vi "Create Plugins.vi"(5 "framework options":T1={"FIFO Options"={"Infinite Timeouts"=FALSE}, "Thread Options"={"Show FP On Call"=FALSE, "Close FP After Call"=FALSE, "Allow Debugging"=FALSE}, "Plugin Options"={"Default Components"=FALSE}, "Performance Options"={"Measure Period"=FALSE, "Measure Rx/Tx Duration"=FALSE}, "Data Server Options"={"Enable Data Server"=FALSE, "Period"=50}} {"Data Server Options"."Period" format="%d ms"}, 7 "framework configuration":T7, 8 "error in (no error)":errorcluster, 10 "components directory":path, 11 "Framework in":refnum<class "Framework.lvclass">) -> (0 "error out":errorcluster, 1 "Plugin Threads":refnum<class "Plugin Thread.lvclass">[](array[class]), 2 "Plugins":refnum<class "Plugin.lvclass">[](array[class]), 3 "Framework out":refnum<class "Framework.lvclass">)   [LabVIEW 2017, in "DSF Core.lvlib" / "Framework.lvclass"]
uses:
  Framework.lvclass
  Plugin/Plugin.lvclass
  Typedefs/DSF Engine Framework Configuration.ctl
  Typedefs/DSF Engine Plugin Configuration.ctl
  Typedefs/DSF Timing Info.ctl
  Typedefs/DSF Engine Plugin Thread Configuration.ctl
  Typedefs/DSF Settings Info.ctl
  Typedefs/DSF Engine Transfer Group Configuration.ctl
  Typedefs/DSF Direction.ctl
  Typedefs/DSF Engine Transfer Configuration.ctl
  Typedefs/DSF Byte Order.ctl
  Typedefs/DSF Engine Channel Configuration.ctl
  Typedefs/DSF Data Type.ctl
  Typedefs/DSF Timeout Behavior.ctl
  Thread/Plugin/Plugin Thread.lvclass
  Framework Options.ctl
  Typedefs/DSF FIFO Options.ctl
  Thread/Thread Options.ctl
  Typedefs/DSF Plugin Options.ctl
  Typedefs/DSF Performance Options.ctl
  Data Server Options.ctl
  Transceiver/Transceiver.lvclass
  Buffer Converter/Buffer Converter.lvclass
  Framework.lvclass/Framework.ctl
  Configuration/Transfer Group Count (Plugin).vi
  Configuration/Required Buffer Size (Plugin).vi
  Component Loader/Component Loader.lvclass
  Configuration/Configuration Session.lvclass
  Buffers/Buffers.lvclass
  Status/Status Pointer.lvclass
  Framework Status/Framework Status.lvclass
  DSF Core.lvlib
  Thread/Thread.lvclass
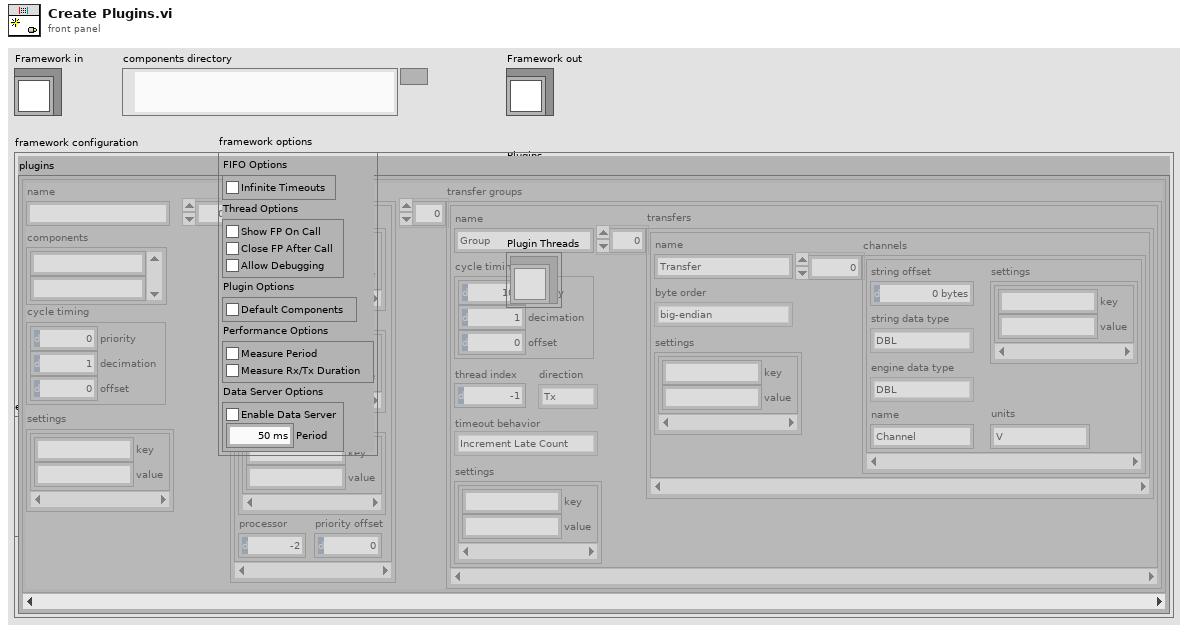
[diagram p1: front panel]
types:
  T1 = typedef "DSF Core.lvlib/Framework.lvclass/Framework Options.ctl" = cluster{"FIFO Options":T2, "Thread Options":T3, "Plugin Options":T4, "Performance Options":T5, "Data Server Options":T6}
  T2 = typedef "DSF Core.lvlib/Framework.lvclass/DSF FIFO Options.ctl" = cluster{"Infinite Timeouts":bool}
  T3 = typedef "DSF Core.lvlib/Thread.lvclass/Thread Options.ctl" = cluster{"Show FP On Call":bool, "Close FP After Call":bool, "Allow Debugging":bool}
  T4 = typedef "DSF Core.lvlib/Framework.lvclass/DSF Plugin Options.ctl" = cluster{"Default Components":bool}
  T5 = typedef "DSF Core.lvlib/DSF Performance Options.ctl" = cluster{"Measure Period":bool, "Measure Rx/Tx Duration":bool}
  T6 = typedef "DSF Core.lvlib/Framework.lvclass/Data Server Options.ctl" = cluster{"Enable Data Server":bool, "Period":u32}
  T7 = typedef "DSF Core.lvlib/DSF Engine Framework Configuration.ctl" = cluster{"plugins":T8[]}
  T8 = typedef "DSF Core.lvlib/DSF Engine Plugin Configuration.ctl" = cluster{"name":string, "components":string[], "cycle timing":T9, "threads":T10[], "transfer groups":T12[], "settings":T11}
  T9 = typedef "DSF Core.lvlib/DSF Timing Info.ctl" = cluster{"priority":u64, "decimation":u64, "offset":u64}
  T10 = typedef "DSF Core.lvlib/DSF Engine Plugin Thread Configuration.ctl" = cluster{"buffer converter settings":T11, "transceiver settings":T11, "custom settings":T11, "processor":i32, "priority offset":i16}
  T11 = typedef "DSF Core.lvlib/DSF Settings Info.ctl" = cluster{"key":string, "value":string}[]
  T12 = typedef "DSF Core.lvlib/DSF Engine Transfer Group Configuration.ctl" = cluster{"name":string, "direction":T13, "cycle timing":T9, "thread index":i32, "settings":T11, "transfers":T14[], "timeout behavior":T18}
  T13 = typedef "DSF Core.lvlib/DSF Direction.ctl" = enum8{"Tx", "Rx"}
  T14 = typedef "DSF Core.lvlib/DSF Engine Transfer Configuration.ctl" = cluster{"name":string, "byte order":T15, "settings":T11, "channels":T16[]}
  T15 = typedef "DSF Core.lvlib/DSF Byte Order.ctl" = enum8{"big-endian", "little-endian"}
  T16 = typedef "DSF Core.lvlib/DSF Engine Channel Configuration.ctl" = cluster{"string offset":u64, "string data type":T17, "engine data type":T17, "name":string, "settings":T11, "units":string}
  T17 = typedef "DSF Core.lvlib/DSF Data Type.ctl" = enum8{"Bool", "SGL", "DBL", "I8", "I16", "I32", "I64", "U8", "U16", "U32", "U64"}
  T18 = typedef "DSF Core.lvlib/DSF Timeout Behavior.ctl" = enum8{"Increment Late Count", "Throw Error"}
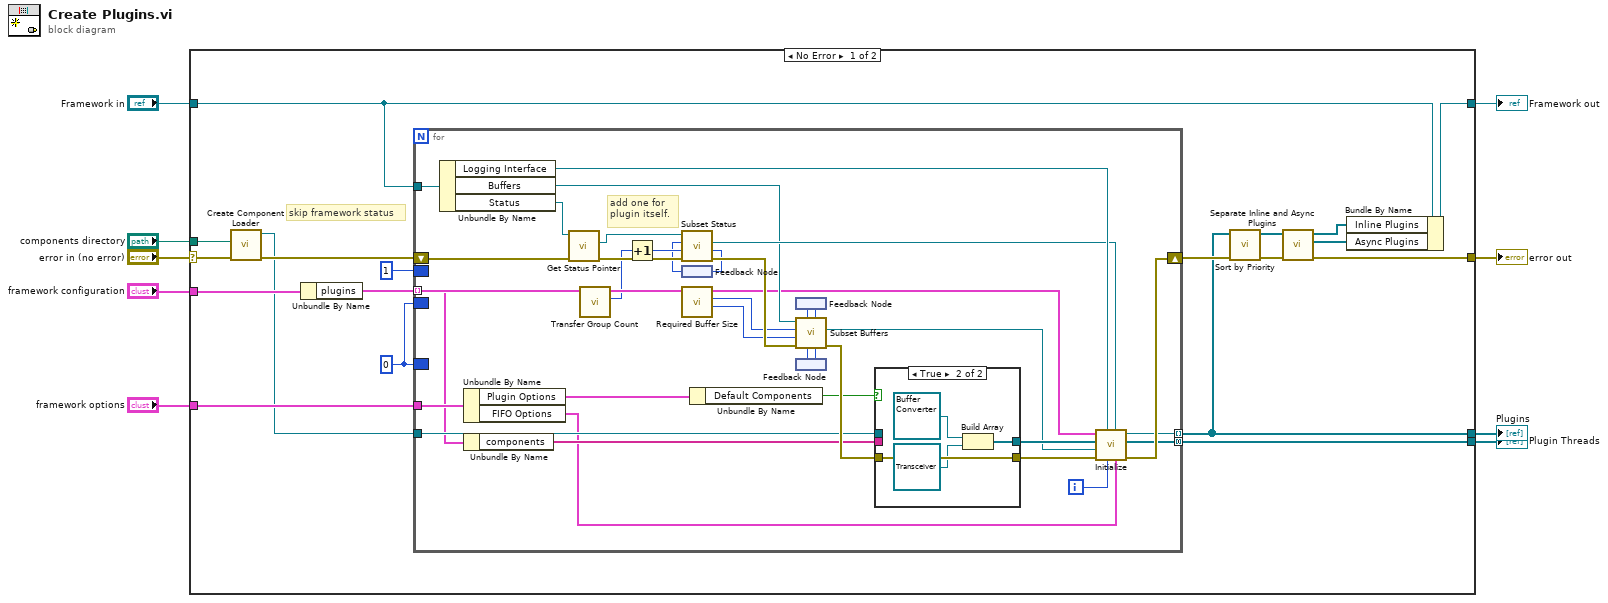
[diagram p0: block diagram]
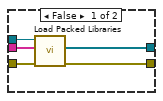
[diagram p2: hidden frame]
diagram:
  n1 = case shown="No Error" "error in (no error)" {
    selector: "error in (no error)" -> [w16 w74]
    tunnel: [w26 w74] -> w9
    tunnel: "framework configuration" -> [w25 _]
    tunnel: [w24 _] -> w7
    tunnel: [w11 _] -> w6
    tunnel: [w20 w75] -> w5
    tunnel: "framework options" -> [w19 _]
    tunnel: "Framework in" -> [w13 w75]
    tunnel: "components directory" -> [w17 _]
    frame No Error {
      w14 = u64 0 ("string buffer offset + size")
      # "skip framework status"
      # "Create Plugins\nIterates through the Plugin configuration clusters to do the following:\n1. Load Plugin components - Uses the Component Loader class to load an array of objects from the Plugin's configured components (PPLs).\n2. Subset Buffers - Subsets the Framework's Buffers to create a set of Buffers for this Plugin and its Transfer Groups and Transfers to use.\n3. Initialize Plugin - Takes the Plugin's subset Buffers and component objects to initialize the Plugin and its Plugin Threads.\n4. Sort and Split Plugins - Sort Plugins by priority to ensure the highest priority Plugins execute first each cycle."
      n2 = call "Create Component Loader.vi"("error in (no error)"=w16, "components directory (default)"=w17) -> ("error out"=w28:errorcluster, "Component Loader out"=w12:refnum<class "Component Loader.lvclass">)  [unwired: 8 in]
      n3 = Unbundle By Name(w25) -> ("plugins"=w15:T8[])
      n4 = for {
        shift-right: [w62] -> w27
        shift-left: w28 -> [w35]
        tunnel: w15 -> [w49] mode=indexing
        tunnel: w12 -> [w45]
        tunnel: [w61] -> w11 mode=indexing
        tunnel: [w51] -> w24 mode=concatenating
        border: w14 -> [_]
        border: w14 -> [_]
        tunnel: w19 -> [w54]
        border: u64 1 ("index + count") -> [_]
        tunnel: w13 -> [w46]
        i -> [w40]
        # "add one for plugin itself."
        n5 = Unbundle By Name(w46) -> ("Logging Interface"=w47:refnum<class "Logging Interface.lvclass">, "Buffers"=w30:refnum<class "Buffers.lvclass">, "Status"=w36:refnum<class "Framework Status.lvclass">)
        n6 = Unbundle By Name(w54) -> ("Plugin Options"=w55:T4, "FIFO Options"=w42:T2)
        n7 = call "Get Status Pointer.vi"("error in (no error)"=w35, "Framework Status in"=w36) -> ("error out"=w34:errorcluster, "status pointer"=w32:refnum<class "Status Pointer.lvclass">)  [unwired: 7 in, 1 out]
        n8 = call-poly "Transfer Group Count.vi"("Plugin Configuration in"=w49) -> ("transfer group count"=w33:i32, "Plugin Configuration out"=w44:T8)  [unwired: 8 in, 1 out]
        n9 = Unbundle By Name(w44) -> ("components"=w43:string[])
        n10 = Increment(x=w33) -> (x+1=w39:i32)
        n11 = feedback #1() -> (w31:u64)
        n12 = call "Subset Status.vi"("error in (no error)"=w34, "count (1)"=w39, "index"=w31, "status pointer in"=w32) -> ("error out"=w63:errorcluster, "index + count"=w50:u64, "subset status pointer"=w37:refnum<class "Status Pointer.lvclass">)  [unwired: 4 in, 1 out]
        n13 = feedback-in #1(w50) -> ()
        n14 = call-poly "Required Buffer Size.vi"("Plugin Configuration in"=w44) -> ("total engine buffer size"=w52:u64, "total string buffer size"=w60:u64, "Plugin Configuration out"=w29:T8)  [unwired: 7 in, 1 out]
        n15 = Unbundle By Name(w55) -> ("Default Components"=w53:bool)
        n16 = feedback #2() -> (w58:u64)
        n17 = feedback #3() -> (w56:u64)
        n18 = call "Subset Buffers.vi"("inline buffer offset"=w56, "string buffer offset"=w58, "error in (no error)"=w63, "inline buffer size"=w52, "string buffer size"=w60, "Buffers in"=w30) -> ("error out"=w64:errorcluster, "subset Buffers"=w41:refnum<class "Buffers.lvclass">, "inline buffer offset +size"=w57:u64, "string buffer offset + size"=w59:u64)  [unwired: 1 in, 1 out]
        n19 = feedback-in #2(w59) -> ()
        n20 = feedback-in #3(w57) -> ()
        n21 = case shown="True" w53 {
          tunnel: [w69 w73] -> w38
          tunnel: w45 -> [w68 _]
          tunnel: w64 -> [w67 w73]
          tunnel: w43 -> [w66 _]
          tunnel: [w65 w70] -> w48
          frame False {
            n22 = call "Load Packed Libraries.vi"("error in (no error)"=w67, "packed library names"=w66, "Component Loader in"=w68) -> ("error out"=w69:errorcluster, "objects"=w65:refnum<class>[])  [unwired: 6 in, 1 out]
          }
          frame True {
            n23 = Build Array(refnum<class "Buffer Converter.lvclass"> refnum ("DSF Core.lvlib:Buffer Converter"), refnum<class "Transceiver.lvclass"> refnum ("DSF Core.lvlib:Transceiver")) -> (w70:refnum<class>[])
          }
        }
        n24 = call "Initialize.vi"("FIFO Options"=w42, "Plugin Status Pointer"=w37, "id"=w40, "Logging Interface"=w47, "error in (no error)"=w38, "Plugin Buffers"=w41, "component objects"=w48, "Plugin Configuration"=w29) -> ("error out"=w62:errorcluster, "Plugin Threads"=w51:refnum<class "Plugin Thread.lvclass">[], "Plugin out"=w61:refnum<class "Plugin.lvclass">)  [unwired: 1 in]
      }
      n25 = call "Sort by Priority.vi"("error in (no error)"=w27, "Plugins in"=w11) -> ("error out"=w23:errorcluster, "Plugins out"=w18:refnum<class "Plugin.lvclass">[])  [unwired: 8 in]
      n26 = call "Separate Inline and Async Plugins.vi"("error in (no error)"=w23, "Plugins"=w18) -> ("error out"=w26:errorcluster, "Async Plugins"=w21:refnum<class "Plugin.lvclass">[], "Inline Plugins"=w22:refnum<class "Plugin.lvclass">[])  [unwired: 7 in]
      n27 = Bundle By Name(cluster=w13, "Inline Plugins"=w22, "Async Plugins"=w21) -> (w20:refnum<class "Framework.lvclass">)
    }
    frame Error {
    }
  }
  "error out" <- w9
  "Framework out" <- w5
  "Plugins" <- w6
  "Plugin Threads" <- w7
